vi "Picture Selection.vi"() -> (2 "Valve Pictures":T1={"Command"={"Error"=enum."InError", "Config"=enum."InConfig", "Stale"=enum."InStale", "Close"=enum."InClose", "Open"=enum."InOpen", "TranClose"=enum."Blank", "TranOpen"=enum."Blank"}, "Feedback"={"Error"=enum."OutError", "Config"=enum."OutConfig", "Stale"=enum."OutStale", "Closed"=enum."OutClose", "Open"=enum."OutOpen", "TranClose"=enum."OutTranClose", "TranOpen"=enum."Blank"}, "Energized"={"Error"=enum."EnError", "Config"=enum."EnConfig", "Stale"=enum."EnStale", "False"=enum."EnOff", "True"=enum."EnOn"}})   [LabVIEW 2020, in "VolatusGUI.lvlib" / "2WayValve.lvclass"]
uses:
  2WayValve.lvclass
  2WayValve.lvclass/2WayValve.ctl
  Picture.ctl
  Command Pictures.ctl
  Feedback Pictures.ctl
  Energized Pictures.ctl
  Valve Pictures.ctl
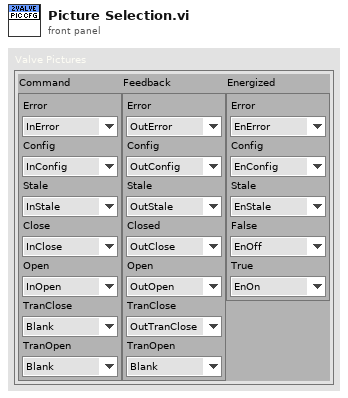
[diagram p1: front panel]
types:
  T1 = typedef "VolatusGUI.lvlib/2WayValve.lvclass/Valve Pictures.ctl" = cluster{"Command":T2, "Feedback":T4, "Energized":T5}
  T2 = typedef "VolatusGUI.lvlib/2WayValve.lvclass/Command Pictures.ctl" = cluster{"Error":T3, "Config":T3, "Stale":T3, "Close":T3, "Open":T3, "TranClose":T3, "TranOpen":T3}
  T3 = typedef "VolatusGUI.lvlib/2WayValve.lvclass/Picture.ctl" = enum16{"Blank", "OutClose", "OutOpen", "OutTranClose", "OutTranOpen", "OutConfig", "OutStale", "OutError", "InClose", "InOpen", "InTranClose", "InTranOpen", "InConfig", "InStale", "InError", "EnOff", "EnOn", "EnConfig", "EnStale", "EnError"}
  T4 = typedef "VolatusGUI.lvlib/2WayValve.lvclass/Feedback Pictures.ctl" = cluster{"Error":T3, "Config":T3, "Stale":T3, "Closed":T3, "Open":T3, "TranClose":T3, "TranOpen":T3}
  T5 = typedef "VolatusGUI.lvlib/2WayValve.lvclass/Energized Pictures.ctl" = cluster{"Error":T3, "Config":T3, "Stale":T3, "False":T3, "True":T3}
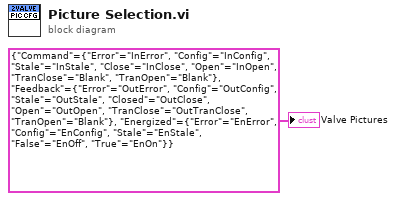
[diagram p0: block diagram]
diagram:
  "Valve Pictures" <- T1 {"Command"={"Error"=enum."InError", "Config"=enum."InConfig", "Stale"=enum."InStale", "Close"=enum."InClose", "Open"=enum."InOpen", "TranClose"=enum."Blank", "TranOpen"=enum."Blank"}, "Feedback"={"Error"=enum."OutError", "Config"=enum."OutConfig", "Stale"=enum."OutStale", "Closed"=enum."OutClose", "Open"=enum."OutOpen", "TranClose"=enum."OutTranClose", "TranOpen"=enum."Blank"}, "Energized"={"Error"=enum."EnError", "Config"=enum."EnConfig", "Stale"=enum."EnStale", "False"=enum."EnOff", "True"=enum."EnOn"}} ("Valve Pictures")
